vi "HDFMixedDataTest.vi"   [LabVIEW 2012]
uses:
  <vilib>/addons/h5labview2/file/H5Fmode.ctl
  <vilib>/addons/h5labview2/base/lib_path.vi
  <vilib>/addons/h5labview2/base/H5Equery.vi
  <vilib>/addons/h5labview2/dataset/H5Dwrite.llb/H5Dwrite.xnode
  <vilib>/addons/h5labview2/file/H5F.lvlib
types:
  T1 = typedef "H5F.lvlib/H5Fmode.ctl" = enum16{"read-only", "read-write", "overwrite", "create new", "open or create"}
  T2 = typedef "hid_t.ctl" = i64
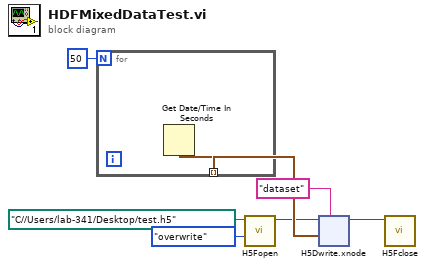
[diagram p0: block diagram]
diagram:
  n1 = for {
    N: 50 -> [_]
    tunnel: [w8] -> w7 mode=indexing
    n2 = Get Date/Time In Seconds() -> (seconds since 1Jan1904=w8:timestamp)
  }
  n3 = call <vilib>:"H5Fopen.vi"("mode (read-only)"=H5Fmode."overwrite", "path"=path "C://Users/lab-341/Desktop/test.h5") -> ("ref out"=w6:T2)  [unwired: 8 in, 1 out]
  n4 = xnode "H5Dwrite.xnode"("dataset name"="dataset", "data"=w7, "ref in"=w6) -> ("ref out"=w5:i64)  [unwired: 4 in, 2 out]
  n5 = call <vilib>:"H5Fclose.vi"("ref"=w5) -> ()  [unwired: 10 in, 1 out]
